vi "QuickSyn_AM_test.vi"() -> ()   [LabVIEW 2017]
uses:
  <userlib>/niRF/niQuickSyn/Core/Properties/RF Frequency/PropertyType.ctl
  <userlib>/niRF/niQuickSyn/Core/Properties/RF Power/PropertyType.ctl
  <userlib>/niRF/niQuickSyn/Core/Properties/AM State/PropertyType.ctl
  <userlib>/niRF/niQuickSyn/Core/Properties/FM Sensitivity/PropertyType.ctl
  <userlib>/niRF/niQuickSyn/Core/Properties/VISA Handle/PropertyType.ctl
  <vilib>/Utility/error.llb/DialogType.ctl
  <userlib>/niRF/niQuickSyn/Core/Properties/RF Output/PropertyType.ctl
  <vilib>/DAQmx/write.llb/DAQmx Write (Analog Wfm 1Chan NSamp).vi
  <vilib>/DAQmx/create/channels.llb/DAQmx Create Channel (AO-Voltage-Basic).vi
  <vilib>/DAQmx/configure/timing.llb/DAQmx Timing (Sample Clock).vi
  <vilib>/DAQmx/miscellaneous.llb/DAQmx Fill In Error Info.vi
  <userlib>/niRF/niQuickSyn/QuickSyn API.lvlib
  <vilib>/measure/NI_MABase.lvlib
  <userlib>/niRF/niQuickSyn/Core/Properties/RF Output/RF Output.lvclass
  <resource>/objmgr/daqmx.rc
  <userlib>/niRF/niQuickSyn/Core/Properties/RF Frequency/RF Frequency.lvclass
  <userlib>/niRF/niQuickSyn/Core/Properties/RF Power/RF Power.lvclass
  <userlib>/niRF/niQuickSyn/Core/Properties/AM State/AM State.lvclass
  <userlib>/niRF/niQuickSyn/Core/Properties/FM Sensitivity/FM Sensitivity.lvclass
  <userlib>/niRF/niQuickSyn/Core/Properties/VISA Handle/VISA Handle.lvclass
panel:
  in  "Stop":bool
  in  "Generator Name":T1="QuickSyn_generator"
  out "Waveform Graph":waveform(dbl)(graph)={"t0"=timestamp(0 s since 1904-01-01), "dt"=2e-06, "Y"=array[50000 elements]}
  in  "AM Depth":T2=100.0 format="%#_9p"
  in  "Amplitude Modulation":T3=enum."Enabled"
  in  "RF Output":bool=TRUE
  in  "error in (no error)":errorcluster
  out "AO.Max":dbl=1.0
  out "AO.Min":dbl=-1.0
  out "error out":errorcluster
  in  "AO max":dbl=1.0 format="%0.2f"
  in  "RF Power, dB":T4=5.0
  in  "RF Frequency, Hz":T5=200000000.0 format="%#_9p"
  in  "Modulation frequency, Hz":dbl=10000.0 format="%0.1p"
  in  "Modulation amplitude, V":dbl=0.5 format="%0.3f"
  in  "AO channel":tag="DAQ6363/ao0"
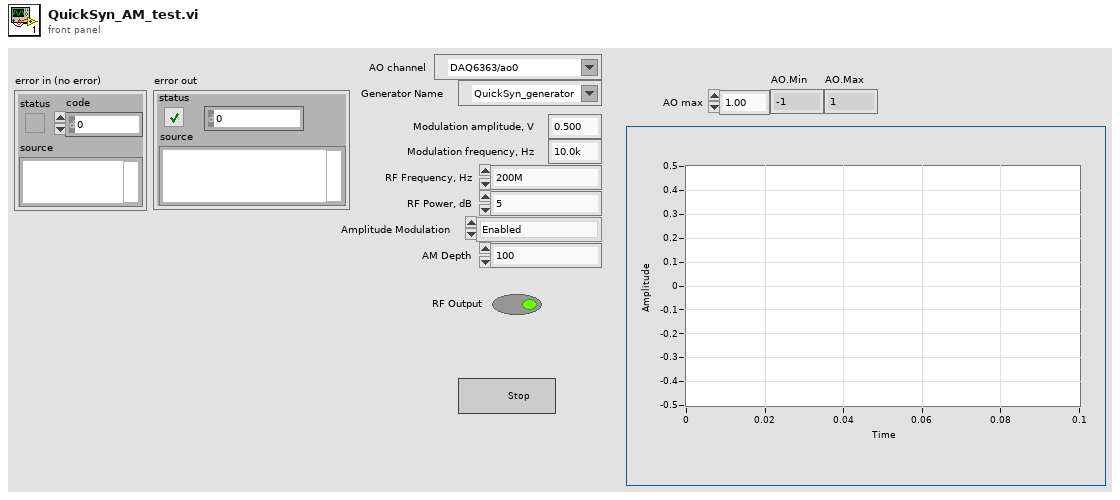
[diagram p1: front panel]
types:
  T1 = typedef "QuickSyn API.lvlib/VISA Handle.lvclass/PropertyType.ctl" = refnum<visa-resource-name>
  T2 = typedef "QuickSyn API.lvlib/FM Sensitivity.lvclass/PropertyType.ctl" = dbl
  T3 = typedef "QuickSyn API.lvlib/AM State.lvclass/PropertyType.ctl" = enum16{"Disabled", "Enabled"}
  T4 = typedef "QuickSyn API.lvlib/RF Power.lvclass/PropertyType.ctl" = dbl
  T5 = typedef "QuickSyn API.lvlib/RF Frequency.lvclass/PropertyType.ctl" = dbl
  T6 = typedef "QuickSyn API.lvlib/RF Output.lvclass/PropertyType.ctl" = bool
  T7 = typedef "DialogType.ctl" = u16
  T8 = enum16{"Sine Wave", "Triangle Wave", "Square Wave", "Sawtooth Wave"}
  T9 = typedef "QuickSyn API.lvlib/QuickSyn.lvclass/Session Handle.ctl" = refnum<data-value>
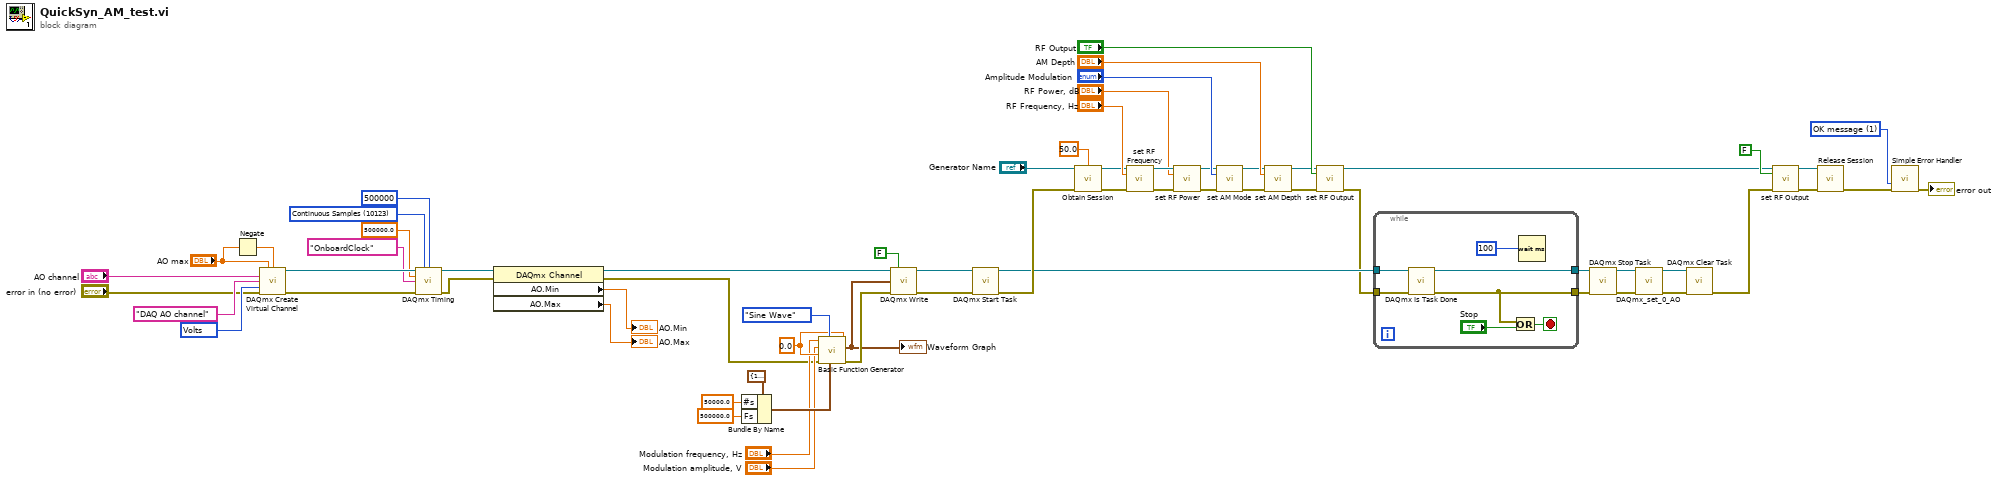
[diagram p0: block diagram]
diagram:
  w32 = 10123 items=["Finite Samples"=10178, "Continuous Samples"=10123, "Hardware Timed Single Point"=12522] ("sample mode")
  w45 = T7 1 items=["no dialog", "OK message", "continue or stop message", "OK message + warnings", "continue/stop + warnings"] ("type of dialog (OK msg:1)")
  w54 = 0.0 ("phase")
  w65 = 10348 items=["Volts"=10348, "From Custom Scale"=10065] ("units")
  n1 = Negate(x="AO max") -> (-x=w47:dbl)
  n2 = call-poly <vilib>:"DAQmx Create Virtual Channel.vi"("maximum value"="AO max", "minimum value"=w47, "physical channels"="AO channel", "name to assign"="DAQ AO channel", "units"=w65, "error in"="error in (no error)") -> ("task out"=w36:refnum<k21>, "error out"=w35:errorcluster)  [unwired: 8 in]
  n3 = call-poly <vilib>:"DAQmx Timing.vi"("task/channels in"=w36, "sample mode"=w32, "samples per channel"=500000, "rate"=500000.0, "source"=tag "OnboardClock", "error in"=w35) -> ("task out"=w33:refnum<k21>, "error out"=w34:errorcluster)  [unwired: 8 in]
  n4 = property class="DAQmx Channel"(reference=w33, error in=w34) -> (reference out=w44:refnum<k21>, error out=w26:errorcluster, "AO.Min"=→"AO.Min":dbl, "AO.Max"=→"AO.Max":dbl)
  n5 = Bundle By Name(cluster=cluster{"Fs":dbl, "#s":dbl} {"Fs"=1000.0, "#s"=1000.0} ("sampling info"), "#s"=50000.0, "Fs"=500000.0) -> (w56:cluster{"Fs":dbl, "#s":dbl})
  n6 = call <vilib>:"Basic Function Generator.vi"("offset"=w54, "sampling info"=w56, "signal type"=T8."Sine Wave", "error in (no error)"=w26, "phase"=w54, "amplitude"="Modulation amplitude, V", "frequency"="Modulation frequency, Hz") -> ("error out"=w28:errorcluster, "signal out"=w22:waveform(dbl))  [unwired: 2 in, 1 out]
  "Waveform Graph" <- w22
  n7 = call-poly <vilib>:"DAQmx Write.vi"("task/channels in"=w44, "auto start"=FALSE, "data"=w22, "error in"=w28) -> ("task out"=w49:refnum<k21>, "error out"=w23:errorcluster)  [unwired: 9 in, 1 out]
  n8 = call <vilib>:"DAQmx Start Task.vi"("task/channels in"=w49, "error in"=w23) -> ("task out"=w17:refnum<k21>, "error out"=w20:errorcluster)  [unwired: 12 in]
  n9 = call <userlib>:"Obtain Session.vi"("VISA resource name"="Generator Name", "Serial Timeout"=50.0, "error in (no error)"=w20) -> ("Session Handle"=w27:T9, "error out"=w21:errorcluster)  [unwired: 11 in]
  n10 = call <userlib>:"set RF Frequency.vi"("Session Handle in"=w27, "RF Frequency, Hz (200M)"="RF Frequency, Hz", "error in (no error)"=w21) -> ("Session Handle out"=w62:T9, "error out"=w61:errorcluster)  [unwired: 11 in]
  n11 = call <userlib>:"set RF Power.vi"("Session Handle in"=w62, "RF Power, dB (0)"="RF Power, dB", "error in (no error)"=w61) -> ("Session Handle out"=w6:T9, "error out"=w5:errorcluster)  [unwired: 11 in]
  n12 = call <userlib>:"set AM Mode.vi"("Session Handle in"=w6, "AM State"="Amplitude Modulation", "error in (no error)"=w5) -> ("Session Handle out"=w13:T9, "error out"=w12:errorcluster)  [unwired: 11 in]
  n13 = call <userlib>:"set AM Depth.vi"("Session Handle in"=w13, "AM Depth"="AM Depth", "error in (no error)"=w12) -> ("Session Handle out"=w10:T9, "error out"=w8:errorcluster)  [unwired: 11 in]
  n14 = call <userlib>:"set RF Output.vi"("Session Handle in"=w10, "RF Output (False)"="RF Output", "error in (no error)"=w8) -> ("Session Handle out"=w9:T9, "error out"=w7:errorcluster)  [unwired: 11 in]
  n15 = while {
    tunnel: w17 -> [w72]
    tunnel: w7 -> [w71]
    tunnel: [w67] -> w18
    tunnel: [w69] -> w16
    stop <- w70 stop-if-true
    n16 = call <vilib>:"DAQmx Is Task Done.vi"("task/channels in"=w72, "error in"=w71) -> ("task out"=w69:refnum<k21>, "error out"=w67:errorcluster)  [unwired: 11 in, 1 out]
    n17 = Or(x=w67, y="Stop") -> (x .or. y?=w70:bool)
    n18 = Wait (ms)(milliseconds to wait=u32 100 ("millisecond multiple")) -> ()  [unwired: 1 out]
  }
  n19 = call <vilib>:"DAQmx Stop Task.vi"("task/channels in"=w16, "error in"=w18) -> ("task out"=w4:refnum<k21>, "error out"=w3:errorcluster)  [unwired: 12 in]
  n20 = call "DAQmx_set_0_AO.vi"("Refnum in"=w4, "error in (no error)"=w3) -> ("Refnum out"=w2:refnum<k21>, "error out"=w1:errorcluster)  [unwired: 12 in]
  n21 = call <vilib>:"DAQmx Clear Task.vi"("task in"=w2, "error in"=w1) -> ("error out"=w40:errorcluster)  [unwired: 13 in]
  n22 = call <userlib>:"set RF Output.vi"("Session Handle in"=w9, "RF Output (False)"=T6 FALSE, "error in (no error)"=w40) -> ("Session Handle out"=w39:T9, "error out"=w38:errorcluster)  [unwired: 11 in]
  n23 = call <userlib>:"Release Session.vi"("Session Handle"=w39, "error in (no error)"=w38) -> ("error out"=w25:errorcluster)  [unwired: 13 in]
  n24 = call <vilib>:"Simple Error Handler.vi"("type of dialog (OK msg:1)"=w45, "error in (no error)"=w25) -> ("error out"=→"error out":errorcluster)  [unwired: 3 in, 4 out]
